vi "TSM SSC Digital PPMU Source Voltage Per-Site.vi"(0 "Digital TSM In":T1, 5 "Per-Site Source Voltages (V)":dbl[](array[numeric]) format="%#_6p", 7 "Current Limit Range (A)":dbl format="%#_6p", 11 "error in":errorcluster) -> (4 "Digital TSM Out":T1, 15 "error out":errorcluster)   [LabVIEW 2020]
doc: "Sources per-site voltages from the PPMU on all specified pin(s) and pin group(s) connected to each site. This function takes in an array of voltages where rows correspond to sites."
uses:
  TSM/TSM SSC Digital.ctl
  <vilib>/NI_TestStand_SemiconductorModule/NI_TestStand_Semiconductor_Module.lvlibp/PinMap/Digital Pattern/PinQueryContext/DigitalPatternPinQueryContext.lvclass
  SSC Digital/SSC Digital.ctl
  <instrlib>/niDigital/niDigital.llb/niDigital Output Function.ctl
  e99f1c10-0623-41e0-9d1e-049a8a523c3a.vi
  Shared SubVIs/Site List to Site Numbers.vi
  Shared SubVIs/Channel List to Pins.vi
  Shared SubVIs/Trim Whitespace [Inlined].vi
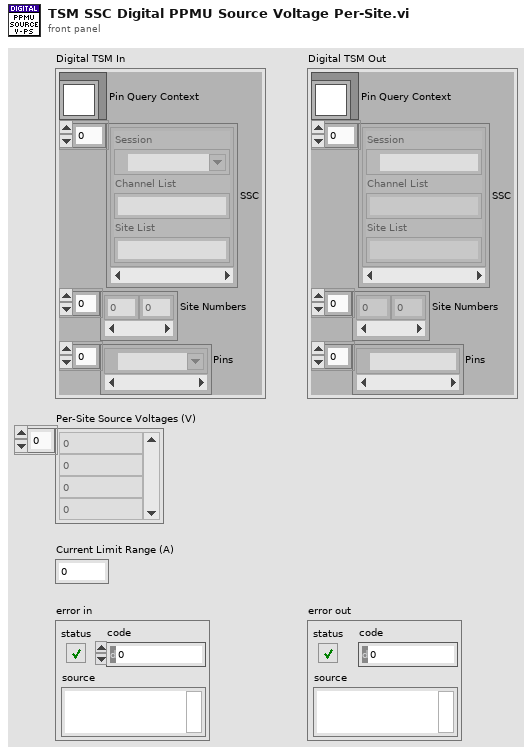
[diagram p1: front panel]
types:
  T1 = typedef "TSM SSC Digital.ctl" = cluster{"Pin Query Context":refnum<class "DigitalPatternPinQueryContext.lvclass">, "SSC":T2[], "Site Numbers":i32[], "Pins":tag[]}
  T2 = typedef "SSC Digital.ctl" = cluster{"Session":refnum<k15>, "Channel List":string, "Site List":string}
  T3 = typedef "Digital 2D Location.ctl" = cluster{"Row":i32, "Col":i32}
  T4 = typedef "niDigital Output Function.ctl" = i32
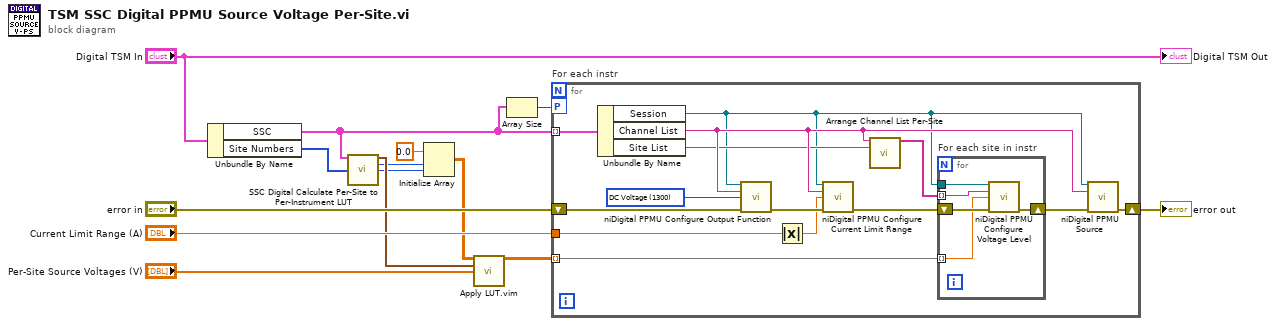
[diagram p0: block diagram]
diagram:
  n1 = Unbundle By Name("Digital TSM In") -> ("SSC"=w1:T2[], "Site Numbers"=w6:i32[])
  n2 = call "SSC Digital Calculate Per-Site to Per-Instrument LUT.vi"("Digital SSC In"=w1, "Sites"=w6) -> ("Per-Site to Per-Instrument LUT"=w8:T3[], "Instrument Count"=w4:i32, "Max Sites on Instrument"=w3:i32)  [unwired: 11 in]
  n3 = Initialize Array(0.0 ("element"), w4, w3) -> (w10:dbl[][])
  n4 = call "Apply LUT.vim"("Initialized Array"=w10, "LUT"=w8, "Results to Apply LUT to"="Per-Site Source Voltages (V)") -> ("Array Out"=w5:dbl[][])  [unwired: 12 in]
  n5 = Array Size(array=w1) -> (size(s)=w2:i32)
  n6 = for "For each instr" {
    tunnel: "Current Limit Range (A)" -> [w27]
    workers-P: w2 -> [_]
    tunnel: w1 -> [w19] mode=indexing
    tunnel: w5 -> [w16] mode=indexing
    shift-right: [w26] -> w14
    shift-left: "error in" -> [w28]
    w23 = T4 1300 items=["DC Voltage"=1300, "DC Current"=1301] ("output function")
    n7 = Unbundle By Name(w19) -> ("Session"=w15:refnum<k15>, "Channel List"=w18:string, "Site List"=w17:string)
    n8 = call <instrlib>:"niDigital PPMU Configure Output Function.vi"("instrument handle"=w15, "channel list"=w18, "output function"=w23, "error in"=w28) -> ("error out"=w25:errorcluster)  [unwired: 10 in, 1 out]
    n9 = Absolute Value(x=w27) -> (abs(x)=w22:dbl)
    n10 = call <instrlib>:"niDigital PPMU Configure Current Limit Range.vi"("instrument handle"=w15, "channel list"=w18, "current limit range (A)"=w22, "error in"=w25) -> ("error out"=w24:errorcluster)  [unwired: 10 in, 1 out]
    n11 = call "Arrange Channel List Per-Site.vi"("Channel List String"=w18, "Site List String"=w17) -> ("Channel List Array"=w20:string[])  [unwired: 11 in, 2 out]
    n12 = for "For each site in instr" {
      tunnel: w20 -> [w33] mode=indexing
      shift-right: [w30] -> w21
      shift-left: w24 -> [w32]
      tunnel: w16 -> [w29] mode=indexing
      tunnel: w15 -> [w31]
      n13 = call <instrlib>:"niDigital PPMU Configure Voltage Level.vi"("instrument handle"=w31, "channel list"=w33, "voltage level (V)"=w29, "error in"=w32) -> ("error out"=w30:errorcluster)  [unwired: 10 in, 1 out]
    }
    n14 = call <instrlib>:"niDigital PPMU Source.vi"("instrument handle"=w15, "channel list"=w18, "error in"=w21) -> ("error out"=w26:errorcluster)  [unwired: 11 in, 1 out]
  }
  "error out" <- w14
  "Digital TSM Out" <- "Digital TSM In"
